vi "Read 2DPictureRef.vi"(8 "error in (no error)":errorcluster, 11 "2DPictureControl in":refnum<class "2DPictureControl.lvclass">=refnum) -> (0 "error out":errorcluster, 2 "2DPictureRef":refnum<vi>, 3 "2DPictureControl out":refnum<class "2DPictureControl.lvclass">)   [LabVIEW 2020, in "2DPictureControl.lvclass"]
uses:
  2DPictureControl.lvclass
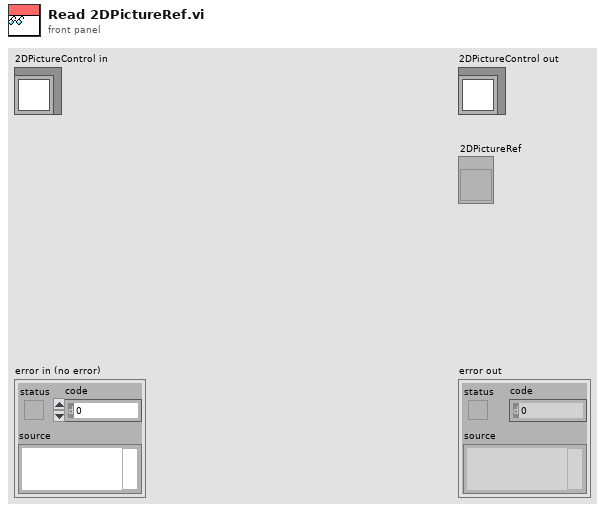
[diagram p1: front panel]
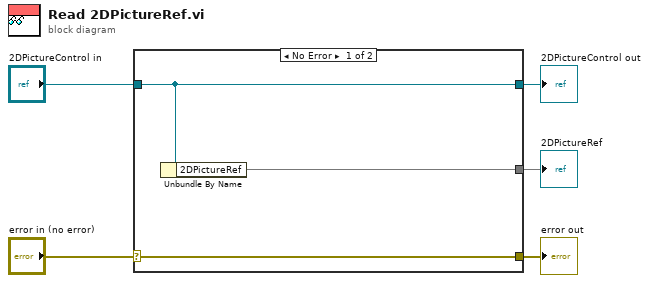
[diagram p0: block diagram]
diagram:
  n1 = case shown="No Error" "error in (no error)" {
    selector: "error in (no error)" -> [w8 w9]
    tunnel: [w8 w9] -> w4
    tunnel: [w7 w10] -> w2
    tunnel: "2DPictureControl in" -> [w7 w10]
    tunnel: [w6 _] -> w1
    frame No Error {
      n2 = Unbundle By Name(w7) -> ("2DPictureRef"=w6)
    }
    frame Error {
    }
  }
  "error out" <- w4
  "2DPictureControl out" <- w2
  "2DPictureRef" <- w1
